vi "IR_LearnEventExe.vi"(0 "Devices In":u64[](array[numeric]), 5 "Event Registration Refnum In":refnum<event-registration>, 11 "error in (no error)":errorcluster) -> (2 "Index":i32, 3 "Event?":bool, 4 "Devices Out":u64[](array[numeric]), 6 "Event Registration Refnum Out":refnum<event-registration>, 8 "Code String":string caption="Code", 10 "codeInfo":T1={"bitCount"=0, "encoding"=1, "length"=1, "gap"=0, "trail"=0, "header[0]"=0, "header[1]"=0, "one[0]"=0, "one[1]"=0, "zero[0]"=0, "zero[1]"=0, "repeat[0]"=0, "repeat[1]"=0, "repeat[2]"=0, "repeat[3]"=0, "repeat[4]"=0, "repeat[5]"=0, "repeat[6]"=0, "repeat[7]"=0, "repeat[8]"=0, "repeat[9]"=0, "repeat[10]"=0, "repeat[11]"=0, "repeat[12]"=0, "repeat[13]"=0, "repeat[14]"=0, "repeat[15]"=0, "repeat[16]"=0, "repeat[17]"=0, "repeat[18]"=0, "repeat[19]"=0, "repeat[20]"=0, "repeat[21]"=0, "repeat[22]"=0, "repeat[23]"=0, "repeat[24]"=0, "repeat[25]"=0, "minRepeat"=0, "dutyCycle"=0.0, "carrierFrequency"=0, "toggleMask[0]"=0, "toggleMask[1]"=0, "toggleMask[2]"=0, "toggleMask[3]"=0, "toggleMask[4]"=0, "toggleMask[5]"=0, "toggleMask[6]"=0, "toggleMask[7]"=0, "toggleMask[8]"=0, "toggleMask[9]"=0, "toggleMask[10]"=0, "toggleMask[11]"=0, "toggleMask[12]"=0, "toggleMask[13]"=0, "toggleMask[14]"=0, "toggleMask[15]"=0, "toggleMask[16]"=0, "toggleMask[17]"=0, "toggleMask[18]"=0, "toggleMask[19]"=0, "toggleMask[20]"=0, "toggleMask[21]"=0, "toggleMask[22]"=0, "toggleMask[23]"=0, "toggleMask[24]"=0, "toggleMask[25]"=0, "toggleMask[26]"=0, "toggleMask[27]"=0, "toggleMask[28]"=0, "toggleMask[29]"=0, "toggleMask[30]"=0, "toggleMask[31]"=0, "toggleMask[32]"=0} {"encoding" items=["IR_ENCODING_UNKNOWN"=1, "IR_ENCODING_SPACE"=2, "IR_ENCODING_PULSE"=3, "IR_ENCODING_BIPHASE"=4, "IR_ENCODING_RC5"=5, "IR_ENCODING_RC6"=6]; "length" items=["IR_LENGTH_UNKNOWN"=1, "IR_LENGTH_CONSTANT"=2, "IR_LENGTH_VARIABLE"=3]}, 14 "phid":u64, 15 "error out":errorcluster)   [LabVIEW 2012, in "Phidget IR.lvlib"]
doc: "${Learn:Header}"
uses:
  <instrlib>/Phidgets/Phidget IR/Phidget IR.lvlib
  <instrlib>/Phidgets/Phidget IR/Public/CodeInfo.ctl
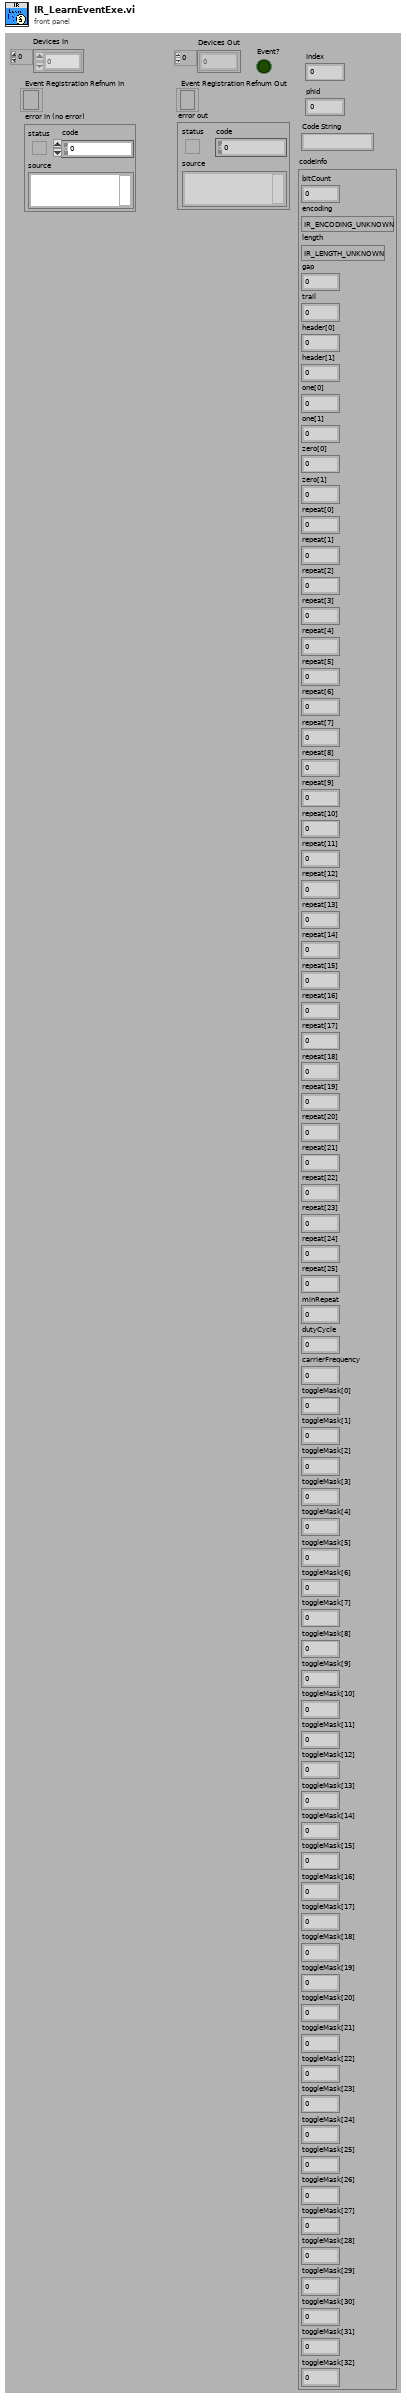
[diagram p1: front panel]
types:
  T1 = typedef "Phidget IR.lvlib/CodeInfo.ctl" = cluster{"bitCount":u32, "encoding":u32, "length":u32, "gap":u32, "trail":u32, "header[0]":u32, "header[1]":u32, "one[0]":u32, "one[1]":u32, "zero[0]":u32, "zero[1]":u32, "repeat[0]":u32, "repeat[1]":u32, "repeat[2]":u32, "repeat[3]":u32, "repeat[4]":u32, "repeat[5]":u32, "repeat[6]":u32, "repeat[7]":u32, "repeat[8]":u32, "repeat[9]":u32, "repeat[10]":u32, "repeat[11]":u32, "repeat[12]":u32, "repeat[13]":u32, "repeat[14]":u32, "repeat[15]":u32, "repeat[16]":u32, "repeat[17]":u32, "repeat[18]":u32, "repeat[19]":u32, "repeat[20]":u32, "repeat[21]":u32, "repeat[22]":u32, "repeat[23]":u32, "repeat[24]":u32, "repeat[25]":u32, "minRepeat":u32, "dutyCycle":dbl, "carrierFrequency":u32, "toggleMask[0]":i8, "toggleMask[1]":i8, "toggleMask[2]":i8, "toggleMask[3]":i8, "toggleMask[4]":i8, "toggleMask[5]":i8, "toggleMask[6]":i8, "toggleMask[7]":i8, "toggleMask[8]":i8, "toggleMask[9]":i8, "toggleMask[10]":i8, "toggleMask[11]":i8, "toggleMask[12]":i8, "toggleMask[13]":i8, "toggleMask[14]":i8, "toggleMask[15]":i8, "toggleMask[16]":i8, "toggleMask[17]":i8, "toggleMask[18]":i8, "toggleMask[19]":i8, "toggleMask[20]":i8, "toggleMask[21]":i8, "toggleMask[22]":i8, "toggleMask[23]":i8, "toggleMask[24]":i8, "toggleMask[25]":i8, "toggleMask[26]":i8, "toggleMask[27]":i8, "toggleMask[28]":i8, "toggleMask[29]":i8, "toggleMask[30]":i8, "toggleMask[31]":i8, "toggleMask[32]":i8}
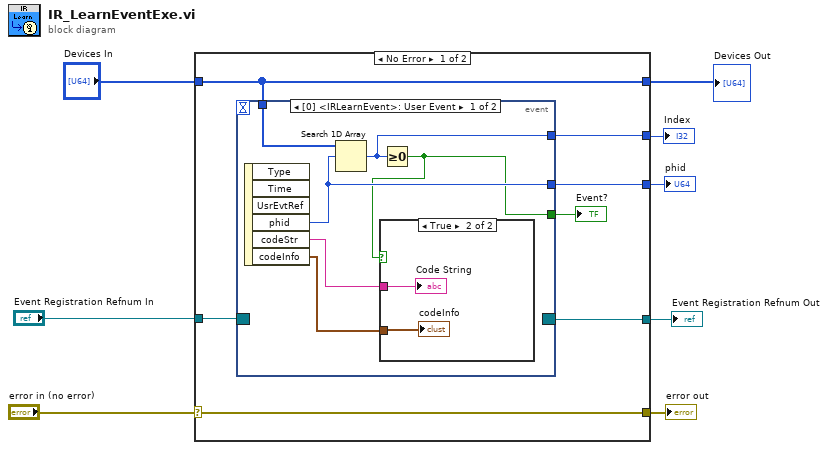
[diagram p0: block diagram]
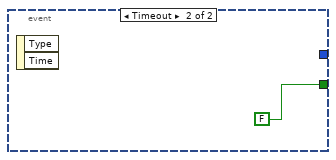
[diagram p3: hidden frame]
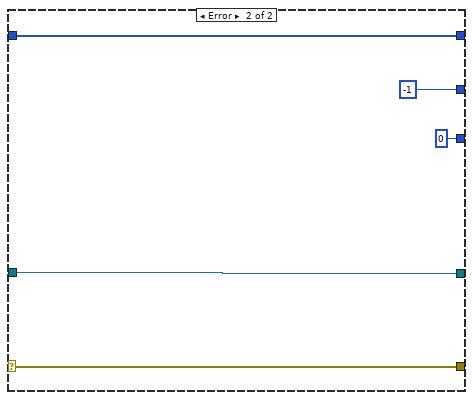
[diagram p4: hidden frame]
diagram:
  n1 = case shown="No Error" "error in (no error)" {
    selector: "error in (no error)" -> [w13 w29]
    tunnel: [w13 w29] -> w7
    tunnel: [w15 w28] -> w2
    tunnel: "Event Registration Refnum In" -> [w14 w28]
    tunnel: [w12 w27] -> w5
    tunnel: "Devices In" -> [w12 w27]
    tunnel: [w11 -1] -> w4
    tunnel: [w10 u64 0 ("phid")] -> w3
    frame No Error {
      n2 = event shown="[0] <IRLearnEvent>: User Event" {
        selector: w14 -> [_ _]
        dyn-events: [_ _] -> w15
        timeout: _ -> [_ _]
        tunnel: w12 -> [w21 _]
        tunnel: [w20 _] -> w11
        tunnel: [w18 _] -> w10
        tunnel: [w17 FALSE] -> w9
        event User Event {
          n3 = event-data() -> ("phid"=w18:u64, "codeStr"=w19:string, "codeInfo"=w16:T1)  [unwired: 1 in, 3 out]
          n4 = Search 1D Array(1D array=w21, element=w18) -> (index of element=w20:i32)  [unwired: 1 in]
          n5 = Greater Or Equal To 0?(x=w20) -> (x >= 0?=w17:bool)
          n6 = case shown="True" w17 {
            tunnel: w19 -> [_ w23]
            tunnel: w16 -> [_ w22]
            frame False {
            }
            frame True {
              "Code String" <- w23
              "codeInfo" <- w22
            }
          }
        }
        event Timeout {
          n7 = event-data() -> ()  [unwired: 1 in, 2 out]
        }
      }
      "Event?" <- w9
    }
    frame Error {
    }
  }
  "error out" <- w7
  "Devices Out" <- w5
  "Index" <- w4
  "phid" <- w3
  "Event Registration Refnum Out" <- w2
